vi "Fail.vi"(7 "Caller":string, 8 "error in (no error)":errorcluster, 9 "Message":string, 10 "Assertion":string, 11 "LVUnit Test Framework in":refnum<class "LVUnit Test Framework.lvclass">) -> (0 "error out":errorcluster, 3 "LVUnit Test Framework out":refnum<class "LVUnit Test Framework.lvclass">)   [LabVIEW 2017, in "Transparent Assertions.lvlib" / "LVUnit Test Framework.lvclass"]
doc: "Executes the unit test framework-specific operation to indicate a failing test."
uses:
  LVUnit Test Framework.lvclass
  Transparent Assertions.lvlib
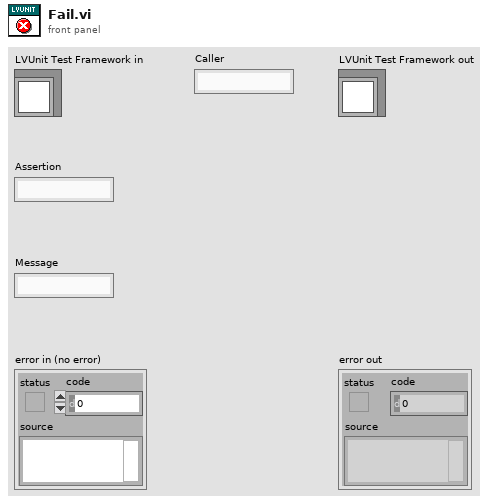
[diagram p1: front panel]
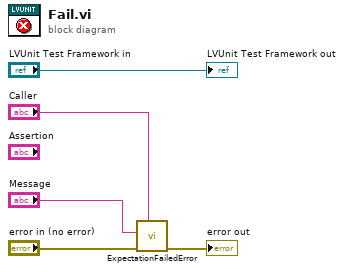
[diagram p0: block diagram]
diagram:
  n1 = call "ExpectationFailedError.vi"("Source (caller)"="Caller", "error in (no error)"="error in (no error)", "Message"="Message") -> ("error out"=→"error out":errorcluster)  [unwired: 8 in]
  "LVUnit Test Framework out" <- "LVUnit Test Framework in"
